vi "STS_Add_Ref_Rawdata.vi"(4 "monitorData":sgl[](array[numeric]), 6 "MPMData":sgl[](array[numeric]), 8 "错误输入（无错误）":errorcluster, 10 "Setting":refnum<k24>, 11 "STSProcess.PDLSTS":refnum<k24>) -> (0 "错误输出":errorcluster, 3 "PDLSTS":refnum<k24>)   [LabVIEW 2017]
uses:
  D:/test/PDLSTS/LV_PDL LvVer17.0/LV_PDL_x86/DLL/STSProcess.dll
  DLL/STSProcess.dll
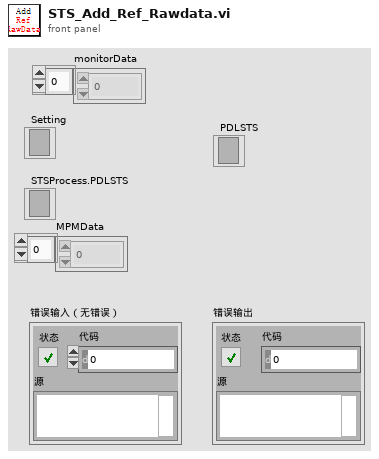
[diagram p1: front panel]
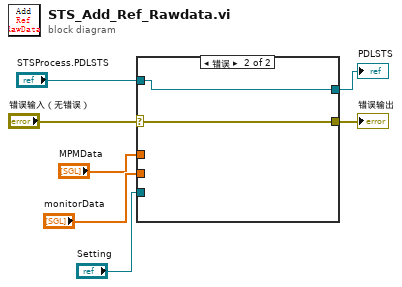
[diagram p0: block diagram]
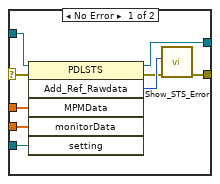
[diagram p2: hidden frame]
diagram:
  n1 = case shown="错误" "错误输入（无错误）" {
    selector: "错误输入（无错误）" -> [w15 w18]
    tunnel: [w11 w18] -> w7
    tunnel: "Setting" -> [w10 _]
    tunnel: "STSProcess.PDLSTS" -> [w16 w17]
    tunnel: [w14 w17] -> w3
    tunnel: "monitorData" -> [w9 _]
    tunnel: "MPMData" -> [w8 _]
    frame No Error {
      n2 = invoke on="调用节点" class="PDLSTS" method="Add_Ref_Rawdata"(reference=w16, error in=w15, "MPMData"=w8, "monitorData"=w9, "setting"=w10) -> (reference out=w14:refnum<k24>, error out=w12:errorcluster, "Add_Ref_Rawdata"=w13:i32)  [unwired: 1 in, 3 out]
      n3 = call "Show_STS_Error.vi"("error in (no error)"=w12, "Error"=w13) -> ("error out"=w11:errorcluster)  [unwired: 9 in]
    }
    frame Error {
    }
  }
  "错误输出" <- w7
  "PDLSTS" <- w3
